vi "写入手动量程.vi"(8 "error in (no error)":errorcluster caption="错误输入（无错误）", 10 "手动量程":dbl(ring)=5.5 items=["4.5"=4.5, "5.5"=5.5, "6.5"=6.5], 11 "数字多用表接口输入":refnum<class "数字多用表接口.lvclass">) -> (0 "error out":errorcluster caption="错误输出", 3 "数字多用表接口输出":refnum<class "数字多用表接口.lvclass">)   [LabVIEW 2020, in "数字多用表接口.lvlib" / "数字多用表接口.lvclass"]
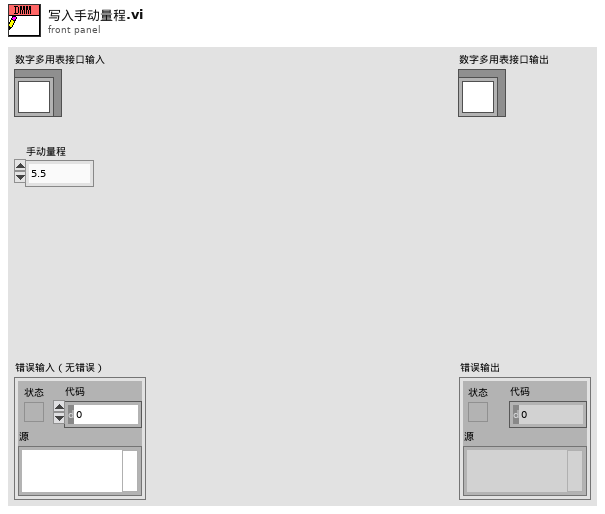
[diagram p1: front panel]
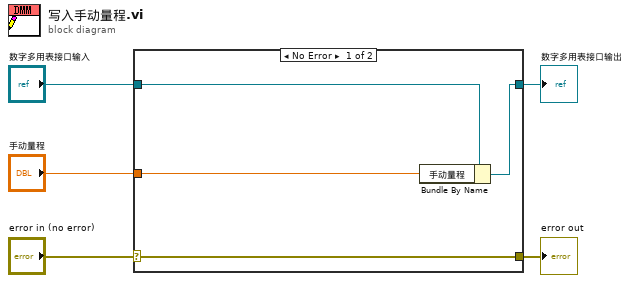
[diagram p0: block diagram]
diagram:
  n1 = case shown="No Error" "error in (no error)" {
    selector: "error in (no error)" -> [w9 w10]
    tunnel: [w9 w10] -> w4
    tunnel: [w7 w11] -> w2
    tunnel: "数字多用表接口输入" -> [w8 w11]
    tunnel: "手动量程" -> [w6 _]
    frame No Error {
      n2 = Bundle By Name(cluster=w8, "手动量程"=w6) -> (w7:refnum<class "数字多用表接口.lvclass">)
    }
    frame Error {
    }
  }
  "error out" <- w4
  "数字多用表接口输出" <- w2
